vi "ams_demo.vi"() -> ()   [LabVIEW 2017]
uses:
  <vilib>/Instr/_visa.llb/VISA Configure Serial Port (Instr).vi
panel:
  out "Histogram":dynamicdata(graph)
  in  "停止按钮":bool
  in  "当前通道":enum32{"模拟通道1", "模拟通道2", "数字通道1", "数字通道2"}(radio) caption="单选按钮"
  out "波形图":dbl[](graph)
  out "当前采样值":dbl(knob) scale=0.0..5.0
  in  "串口号：":refnum<visa-resource-name>
  # "基于Arduino+LabVIEW的多路数据采集系统"
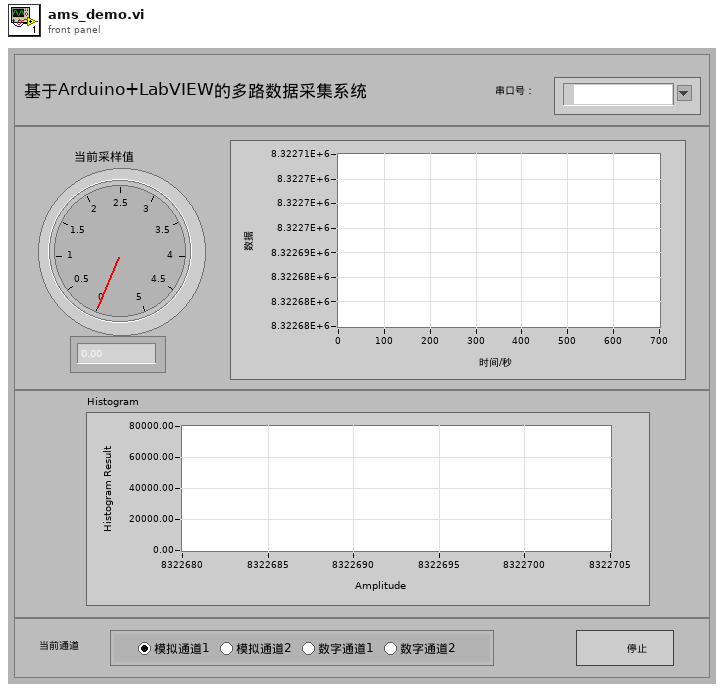
[diagram p1: front panel]
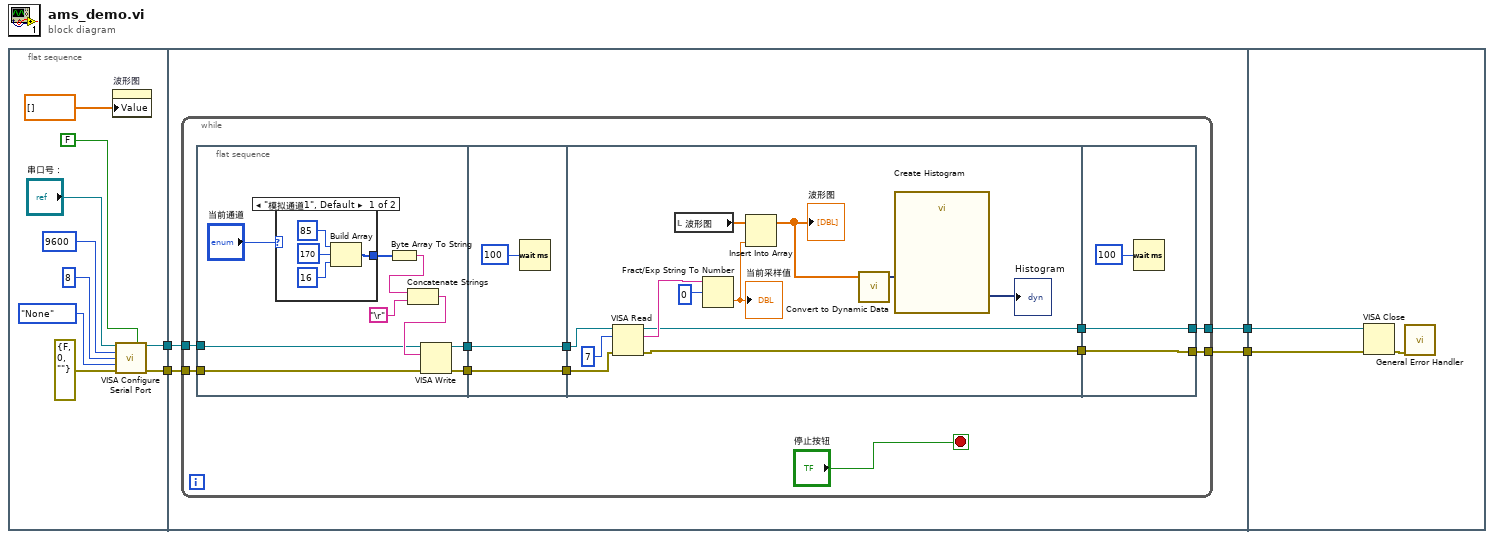
[diagram p0: block diagram]
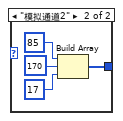
[diagram p2: hidden frame]
diagram:
  n1 = flat-sequence {
    tunnel: [w7] -> w4
    tunnel: [w6] -> w3
    tunnel: w4 -> [w17]
    tunnel: w3 -> [w16]
    tunnel: [w15] -> w2
    tunnel: [w14] -> w1
    tunnel: w2 -> [w65]
    tunnel: w1 -> [w64]
    frame #0 {
      n2 = property on="波形图" class="WFGraph (strict)"("Value"=dbl[] [] ("波形图")) -> ()  [unwired: 2 in, 2 out]
      n3 = call-poly "VISA Configure Serial Port"("VISA resource name"="串口号：", "Enable Termination\nChar (T)"=FALSE ("Enable Termination\nChar (T)"), "baud rate (9600)"=u32 9600, "data bits (8)"=u16 8, "parity (0:none)"=enum16{"None", "Odd", "Even", "Mark", "Space"}."None", "error in (no error)"=errorcluster {"status"=FALSE, "code"=0, "source"=""}) -> ("VISA resource name out"=w7:refnum<visa-resource-name>, "error out"=w6:errorcluster)  [unwired: 1 in, 7 out]
    }
    frame #1 {
      n4 = while {
        tunnel: w17 -> [w24]
        tunnel: w16 -> [w23]
        tunnel: [w20] -> w15
        tunnel: [w18] -> w14
        stop <- "停止按钮" stop-if-true
        n5 = flat-sequence {
          tunnel: [w37] -> w28
          tunnel: [w36] -> w27
          tunnel: w24 -> [w29]
          tunnel: w23 -> [w35]
          tunnel: w28 -> [w48]
          tunnel: w27 -> [w47]
          tunnel: [w48] -> w26
          tunnel: [w47] -> w25
          tunnel: w26 -> [w60]
          tunnel: w25 -> [w59]
          tunnel: [w53] -> w21
          tunnel: [w52] -> w19
          tunnel: w21 -> [w62]
          tunnel: [w62] -> w20
          tunnel: [w61] -> w18
          tunnel: w19 -> [w61]
          frame #0 {
            n6 = case shown="\"模拟通道1\", Default" "当前通道" {
              tunnel: [w38 w42] -> w34
              frame "模拟通道1", Default {
                n7 = Build Array(85, 170, 16) -> (w38:i32[])
              }
              frame "模拟通道2" {
                n8 = Build Array(85, 170, 17) -> (w42:i32[])
              }
            }
            n9 = Byte Array To String(unsigned byte array=w34) -> (string=w33:string)
            n10 = Concatenate Strings(w33, "\r") -> (w30:string)
            n11 = VISA Write(VISA resource name=w29, write buffer=w30, error in (no error)=w35) -> (VISA resource name out=w37:refnum<visa-resource-name>, error out=w36:errorcluster)  [unwired: 1 out]
          }
          frame #1 {
            n12 = Wait (ms)(milliseconds to wait=u32 100 ("等待时间（毫秒）")) -> ()  [unwired: 1 out]
          }
          frame #2 {
            n13 = VISA Read(VISA resource name=w60, byte count=u32 7 ("字节总数"), error in (no error)=w59) -> (VISA resource name out=w53:refnum<visa-resource-name>, read buffer=w56:string, error out=w52:errorcluster)  [unwired: 1 out]
            n14 = local read "波形图"() -> (w55:dbl[])
            n15 = Fract/Exp String To Number(string=w56, offset=0 ("偏移量")) -> (number=w54:dbl)  [unwired: 2 in, 1 out]
            "当前采样值" <- w54
            n16 = Insert Into Array(array=w55, new element=w54) -> (w51:dbl[])  [unwired: 1 in]
            "波形图" <- w51
            n17 = call "Convert to Dynamic Data"("Array"=w51) -> ("Dynamic Data Type"=w50:dynamicdata)  [unwired: 3 in]
            n18 = call "Create Histogram"("Signal"=w50) -> ("Histogram"=→"Histogram":dynamicdata)  [unwired: 9 in, 1 out]
          }
          frame #3 {
            n19 = Wait (ms)(milliseconds to wait=u32 100 ("等待时间（毫秒）")) -> ()  [unwired: 1 out]
          }
        }
      }
    }
    frame #2 {
      n20 = VISA Close(VISA resource name=w65, error in (no error)=w64) -> (error out=w66:errorcluster)
      n21 = call <vilib>:"General Error Handler.vi"("error in (no error)"=w66) -> ()  [unwired: 10 in, 5 out]
    }
  }
